vi "sub_updateSolverArray.vi"(9 "array index":cluster{"row ":i32, "col":i32}, 10 "possible candidates":string[](array[string]), 11 "solver (in)":cluster{"solved":bool, "values":string[]}[][](array[cluster])) -> (3 "solver (out)":cluster{"solved":bool, "values":string[]}[][](array[cluster]))   [LabVIEW 2018]
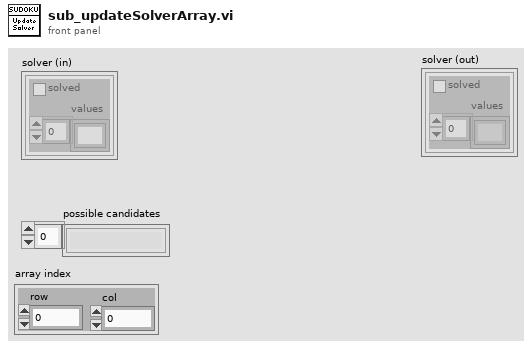
[diagram p1: front panel]
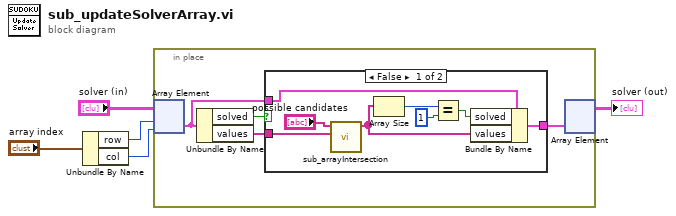
[diagram p0: block diagram]
diagram:
  n1 = Unbundle By Name("array index") -> ("row"=w2:i32, "col"=w1:i32)
  n2 = in-place {
    n3 = in-place-array #1("solver (in)", w2, w1) -> (w8:cluster{"solved":bool, "values":string[]})
    n4 = Unbundle By Name(w8) -> ("solved"=w9:bool, "values"=w6:string[])
    n5 = case shown="False" w9 {
      tunnel: w8 -> [w13 w18]
      tunnel: [w12 w18] -> w7
      tunnel: w6 -> [w11 _]
      frame False {
        n6 = call "sub_arrayIntersection.vi"("set 2"=w11, "set 1"="possible candidates") -> ("set 1  & set 2"=w14:string[])  [unwired: 9 in]
        n7 = Array Size(array=w14) -> (size(s)=w17:i32)
        n8 = Equal?(x=w17, y=1) -> (x = y?=w15:bool)
        n9 = Bundle By Name(cluster=w13, "solved"=w15, "values"=w14) -> (w12:cluster{"solved":bool, "values":string[]})
      }
      frame True {
      }
    }
    n10 = in-place-array #1(w7) -> (→"solver (out)":cluster{"solved":bool, "values":string[]}[][])  [unwired: 2 out]
  }
